vi "CIMAQ_PM_BoundingC.vi"(8 "error in (no error)":errorcluster, 10 "Speedup":i32=1, 11 "Imag in":T1) -> (0 "error out":errorcluster, 1 "Bounding Box":cluster{dbl, dbl, dbl, dbl}, 2 "Radius":dbl, 3 "Center":cluster{i32, i32})   [LabVIEW 2017]
uses:
  <vilib>/vision/Image Controls.llb/IMAQ Image.ctl
  <vilib>/vision/NI_Vision_Development_Module.lvlib
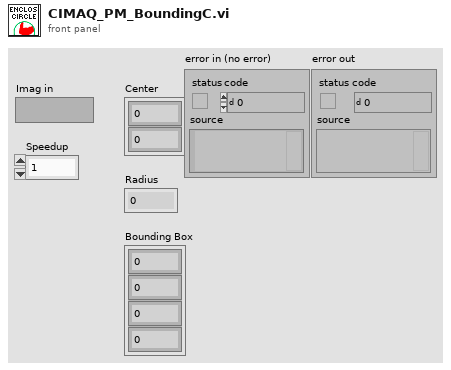
[diagram p1: front panel]
types:
  T1 = typedef "IMAQ Image.ctl" = refnum<image>
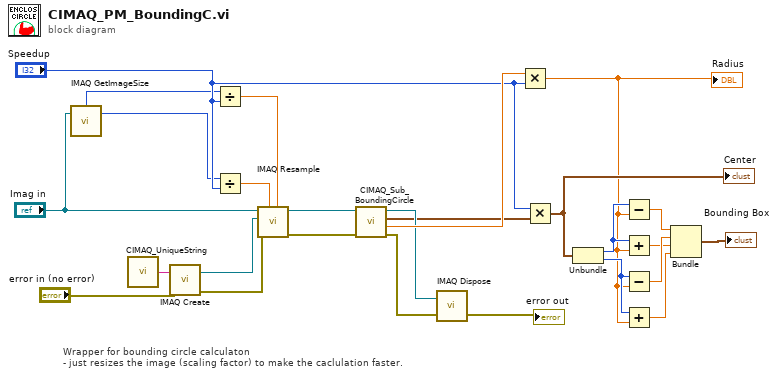
[diagram p0: block diagram]
diagram:
  # "Wrapper for bounding circle calculaton\n- just resizes the image (scaling factor) to make the caclulation faster."
  n1 = call "IMAQ GetImageSize"("Image"="Imag in") -> ("Y Resolution"=w10:i32, "X Resolution"=w9:i32)  [unwired: 3 in, 1 out]
  n2 = call <userlib>:"CIMAQ_UniqueString.vi"() -> ("String"=w16:string)  [unwired: 5 in]
  n3 = call "IMAQ Create"("Image Name"=w16, "error in (no error)"="error in (no error)") -> ("New Image"=w11:T1, "error out"=w5:errorcluster)  [unwired: 3 in]
  n4 = Divide(x=w9, y="Speedup") -> (x/y=w7:dbl)
  n5 = Divide(x=w10, y="Speedup") -> (x/y=w8:dbl)
  n6 = call "IMAQ Resample"("X Resolution"=w7, "Y Resolution"=w8, "error in (no error)"=w5, "Image Dst"=w11, "Image Src"="Imag in") -> ("error out"=w4:errorcluster, "Image Dst Out"=w13:T1)  [unwired: 5 in]
  n7 = call "CIMAQ_Sub_BoundingCircle.vi"("error in (no error)"=w4, "In"=w13) -> ("error out"=w1:errorcluster, "Radius"=w26:dbl, "Center"=w14:cluster{i32, i32}, "Out"=w17:T1)  [unwired: 5 in]
  n8 = call "IMAQ Dispose"("Image"=w17, "error in (no error)"=w1) -> ("error out"=→"error out":errorcluster)  [unwired: 4 in]
  n9 = Multiply(x=w26, y="Speedup") -> (x*y=w3:dbl)
  "Radius" <- w3
  n10 = Multiply(x="Speedup", y=w14) -> (x*y=w25:cluster{i32, i32})
  "Center" <- w25
  n11 = Unbundle(w25) -> (w23:i32, w24:i32)
  n12 = Subtract(x=w23, y=w3) -> (x-y=w22:dbl)
  n13 = Add(x=w23, y=w3) -> (x+y=w20:dbl)
  n14 = Subtract(x=w24, y=w3) -> (x-y=w21:dbl)
  n15 = Add(x=w24, y=w3) -> (x+y=w19:dbl)
  n16 = Bundle(w22, w21, w20, w19) -> (→"Bounding Box":cluster{dbl, dbl, dbl, dbl})  [unwired: 1 in]
